vi "1D Array Stats.vi"(10 "Array":dbl[](array[numeric])) -> (0 "Min":dbl, 1 "Mean":dbl, 2 "Max":dbl, 3 "Relative Standard Deviation":dbl)   [LabVIEW 2016]
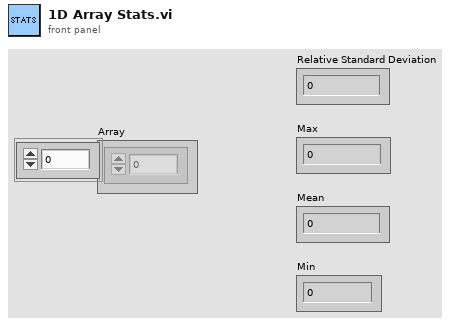
[diagram p1: front panel]
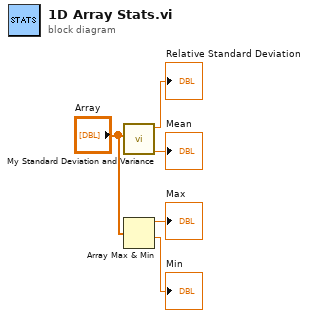
[diagram p0: block diagram]
diagram:
  n1 = call "My Standard Deviation and Variance.vi"("Array - Numeric"="Array") -> ("Mean"=→"Mean":dbl, "Relative Standard Deviation"=→"Relative Standard Deviation":dbl)  [unwired: 7 in, 2 out]
  n2 = Array Max & Min(array="Array") -> (max value=→"Max":dbl, min value=→"Min":dbl)  [unwired: 2 out]
